vi "Pin Map ID Global Variable Name.vi"() -> (0 "global variable name":string="NI.MeasurementLink.PinMapId")   [LabVIEW 2020, in "Measurement Plugin TestStand Integration.lvlib"]
uses:
  Measurement Plugin TestStand Integration.lvlib
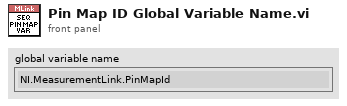
[diagram p1: front panel]
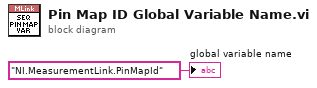
[diagram p0: block diagram]
diagram:
  "global variable name" <- "NI.MeasurementLink.PinMapId" ("lookupString")
